vi "初始化.vi"   [LabVIEW 2018]
types:
  T1 = cluster{"Fx":sgl[], "Fy":sgl[], "Dx":sgl[], "Dy":sgl[]}
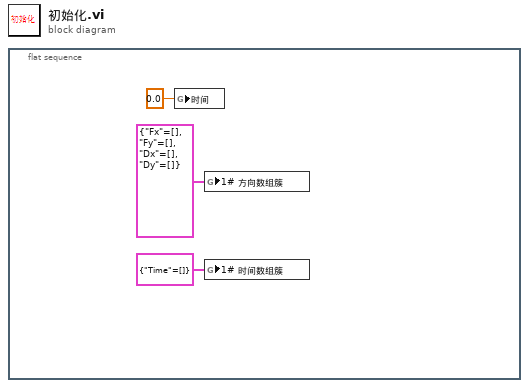
[diagram p0: block diagram]
diagram:
  n1 = flat-sequence {
    frame #0 {
      n2 = global write "全局 1.vi" "时间"(sgl 0.0 ("时间")) -> ()
      n3 = global write "全局 1.vi" "1# 方向数组簇"(T1 {"Fx"=[], "Fy"=[], "Dx"=[], "Dy"=[]} ("1# 方向数组簇")) -> ()
      n4 = global write "全局 1.vi" "1# 时间数组簇"(cluster{"Time":i32[]} {"Time"=[]} ("1# 时间数组簇")) -> ()
    }
  }
